vi "MGCC_FntStaMach_error_classify.vi"(2 "Error":dbl) -> (16 "Error state":bool, 18 "No error":bool)   [LabVIEW 2016]
doc: "-----------------------------------------------------------------------------------------------------------------------\nCopyright <2019> <The University of Tennessee at Knoxville and the University of Tennessee Research Foundation>\nThis software is released under BSD-3 \nhttps://opensource.org/licenses/BSD-3-Clause \nAdditional license options available at https://utrf.tennessee.edu/industry/sample-agreements/\n-----------------------------------------------------------------------------------------------------------------------"
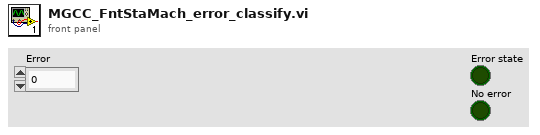
[diagram p1: front panel]
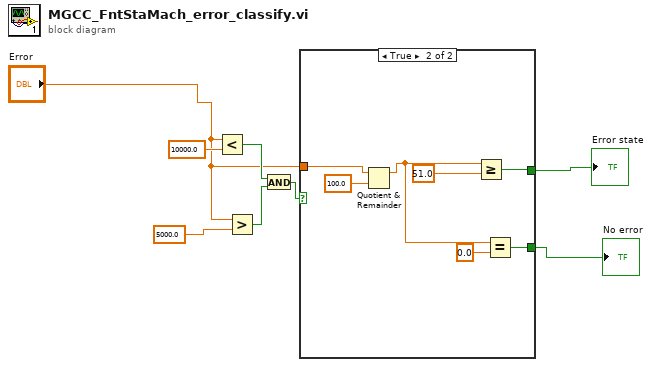
[diagram p0: block diagram]
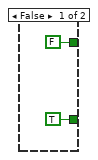
[diagram p2: hidden frame]
diagram:
  n1 = Less?(x="Error", y=10000.0) -> (x < y?=w4:bool)
  n2 = Greater?(x="Error", y=5000.0) -> (0:w3:bool)
  n3 = And(x=w4, y=w3) -> (x .and. y?=w2:bool)
  n4 = case shown="True" w2 {
    tunnel: [FALSE w15] -> w8
    tunnel: [TRUE w12] -> w7
    tunnel: "Error" -> [_ w11]
    frame False {
    }
    frame True {
      n5 = Quotient & Remainder(x=w11, y=100.0) -> (x-y*floor(x/y)=w14:dbl)  [unwired: 1 out]
      n6 = Greater Or Equal?(x=w14, y=51.0) -> (x >= y?=w15:bool)
      n7 = Equal?(x=w14, y=0.0) -> (x = y?=w12:bool)
    }
  }
  "Error state" <- w8
  "No error" <- w7
